vi "Relative2Absolute.vi"(11 "机器人语音指令数据簇":T1) -> (0 "Rot_deg":dbl, 2 "y":dbl, 3 "x":dbl)   [LabVIEW 2014]
uses:
  Global_var/Global_var.vi
  <vilib>/imath/engines/lvmath2/RunTimeEngine/NodeEndStatement/NIMS_NodeEndStatement_Output.vi
  <instcachedir>/0/NIMS_NodeEndStatement_Output_53EC0D466D134D7ABD903AC30B43404B.lvgen/NIMS_NodeEndStatement_Output_53EC0D466D134D7ABD903AC30B43404B_001.vi
  <vilib>/imath/engines/lvmath2/RunTimeEngine/ErrorHandling/NIMS_Finalize Error.vi
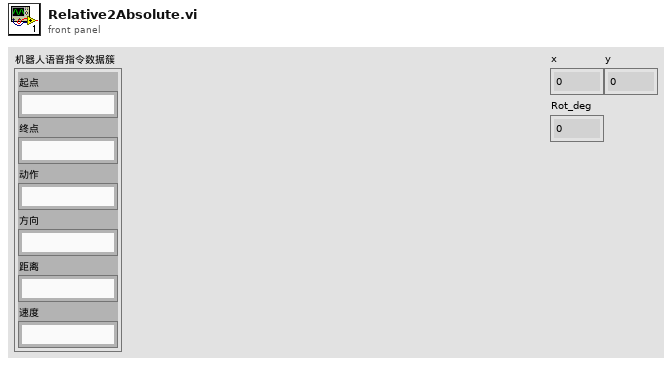
[diagram p1: front panel]
types:
  T1 = cluster{"起点":string, "终点":string, "动作":string, "方向":string, "距离":string, "速度":string}
  T2 = cluster{"now_pose_X":dbl, "now_pose_Y":dbl, "now_pose_Rot_deg":dbl}
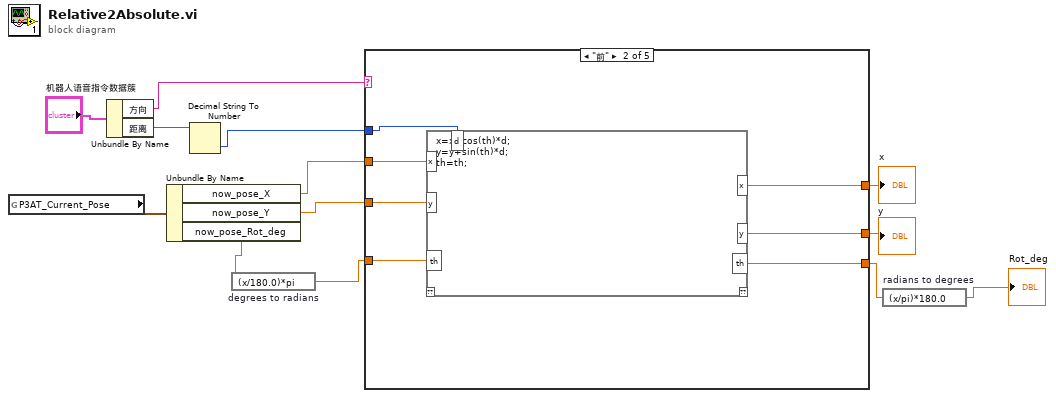
[diagram p0: block diagram]
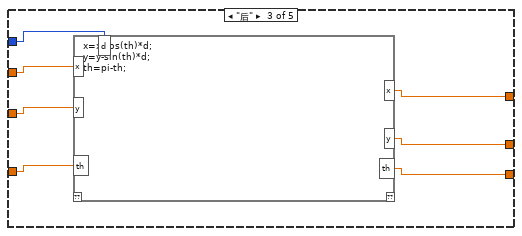
[diagram p3: hidden frame]
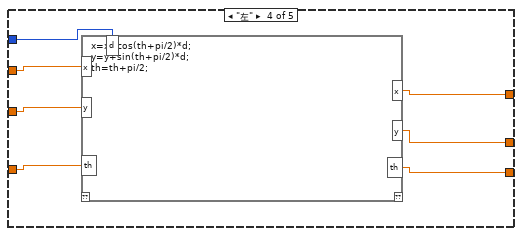
[diagram p4: hidden frame]
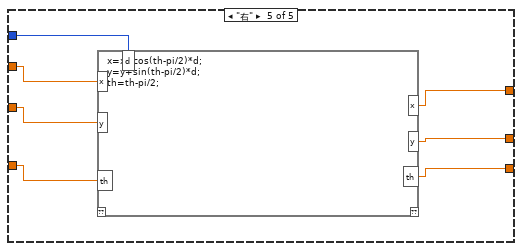
[diagram p5: hidden frame]
diagram:
  n1 = global read "Global_var.vi" "P3AT_Current_Pose"() -> (w13:T2)
  n2 = Unbundle By Name("机器人语音指令数据簇") -> ("方向"=w9:string, "距离"=w8:string)
  n3 = Unbundle By Name(w13) -> ("now_pose_X"=w12:dbl, "now_pose_Y"=w11:dbl, "now_pose_Rot_deg"=w6:dbl)
  n4 = Decimal String To Number(string=w8) -> (number=w7:i32)  [unwired: 2 in, 1 out]
  n5 = expression code="(x/180.0)*pi" "degrees to radians"(w6) -> (w5:dbl)
  n6 = case shown="\"前\"" w9 {
    tunnel: w12 -> [w16 w23 w74 w128 w192]
    tunnel: w11 -> [w15 w22 w73 w127 w191]
    tunnel: w5 -> [w14 w21 w72 w126 w190]
    tunnel: w7 -> [_ w20 w75 w129 w193]
    tunnel: [w16 w19 w71 w125 w189] -> w4
    tunnel: [w15 w18 w70 w124 w188] -> w3
    tunnel: [w14 w17 w69 w123 w187] -> w2
    frame "_", Default {
    }
    frame "前" {
      n7 = mathscript code="x=x+cos(th)*d;\ny=y+sin(th)*d;\nth=th;"("x"=w23, "y"=w22, "th"=w21, "d"=w20) -> ("x"=w19:dbl, "y"=w18:dbl, "th"=w17:dbl)  [unwired: 1 in, 1 out]
    }
    frame "后" {
      n8 = mathscript code="x=x-cos(th)*d;\ny=y-sin(th)*d;\nth=pi-th;"("x"=w74, "y"=w73, "th"=w72, "d"=w75) -> ("x"=w71:dbl, "y"=w70:dbl, "th"=w69:dbl)  [unwired: 1 in, 1 out]
    }
    frame "左" {
      n9 = mathscript code="x=x+cos(th+pi/2)*d;\ny=y+sin(th+pi/2)*d;\nth=th+pi/2;"("x"=w128, "y"=w127, "th"=w126, "d"=w129) -> ("x"=w125:dbl, "y"=w124:dbl, "th"=w123:dbl)  [unwired: 1 in, 1 out]
    }
    frame "右" {
      n10 = mathscript code="x=x+cos(th-pi/2)*d;\ny=y+sin(th-pi/2)*d;\nth=th-pi/2;"("x"=w192, "y"=w191, "th"=w190, "d"=w193) -> ("x"=w189:dbl, "y"=w188:dbl, "th"=w187:dbl)  [unwired: 1 in, 1 out]
    }
  }
  "x" <- w4
  "y" <- w3
  n11 = expression code="(x/pi)*180.0" "radians to degrees"(w2) -> (→"Rot_deg":dbl)
